vi "SinglePointMeasurement.vi"(7 "error out 2":errorcluster, 8 "Measure":T1, 9 "Channel":T2, 10 "VISA resource name 2":refnum<visa-resource-name>) -> (0 "error out":errorcluster, 1 "String":string, 2 "reading":string, 3 "VISA resource name":refnum<visa-resource-name>, 4 "Measuremet":dbl)   [LabVIEW 2021]
uses:
  controls/Channel.ctl
  controls/Measure.ctl
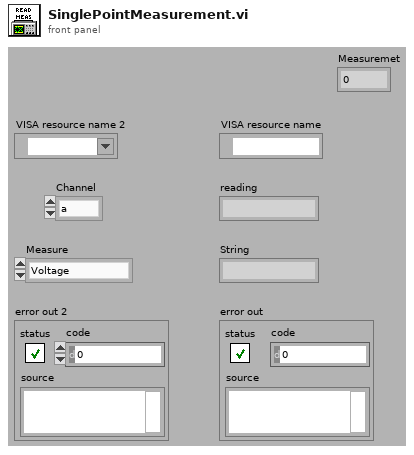
[diagram p1: front panel]
types:
  T1 = typedef "Measure.ctl" = enum16{"Voltage", "Current", "Resistance", "Power"}
  T2 = typedef "Channel.ctl" = enum16{"a", "b"}
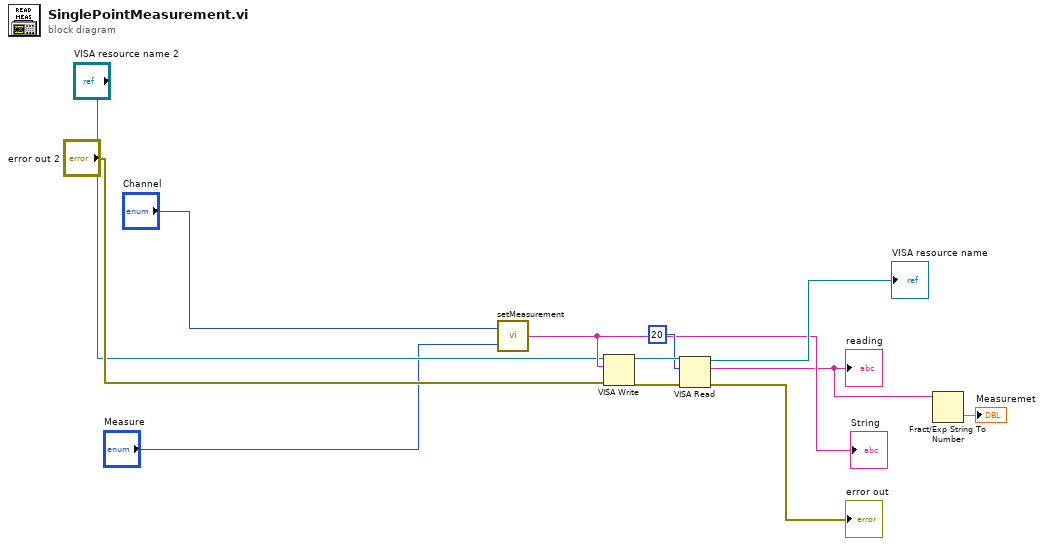
[diagram p0: block diagram]
diagram:
  n1 = call "setMeasurement.vi"("Measure"="Measure", "Channel"="Channel") -> ("String"=w7:string)
  "String" <- w7
  n2 = VISA Write(VISA resource name="VISA resource name 2", write buffer=w7, error in (no error)="error out 2") -> (VISA resource name out=w9:refnum<visa-resource-name>, error out=w10:errorcluster)  [unwired: 1 out]
  n3 = VISA Read(VISA resource name=w9, byte count=u32 20, error in (no error)=w10) -> (VISA resource name out=→"VISA resource name":refnum<visa-resource-name>, read buffer=w2:string, error out=→"error out":errorcluster)  [unwired: 1 out]
  "reading" <- w2
  n4 = Fract/Exp String To Number(string=w2) -> (number=→"Measuremet":dbl)  [unwired: 3 in, 1 out]
